vi "calc power.vi"(11 "Array":dbl[][][](array[numeric])) -> (3 "power":dbl)   [LabVIEW 2015]
panel:
  in  "b":dbl=-4445.0 format="%#_13g"
  in  "k":dbl=0.01138 format="%#_13g"
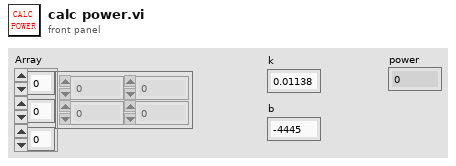
[diagram p1: front panel]
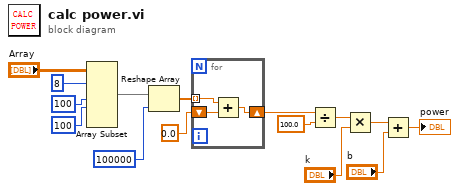
[diagram p0: block diagram]
diagram:
  n1 = Array Subset(array="Array", index (dim 0)=8 ("index"), index (dim 1)=100 ("index"), length (dim 1)=100 ("length")) -> (w1:dbl[][][])  [unwired: 3 in]
  n2 = Reshape Array(w1, 100000 ("dimension size")) -> (w4:dbl[])
  n3 = for {
    tunnel: w4 -> [w18] mode=indexing
    shift-right: [w17] -> w2
    shift-left: 0.0 -> [w16]
    n4 = Add(x=w18, y=w16) -> (x+y=w17:dbl)
  }
  n5 = Divide(x=w2, y=100.0) -> (x/y=w6:dbl)
  n6 = Multiply(x=w6, y="k") -> (x*y=w14:dbl)
  n7 = Add(x=w14, y="b") -> (x+y=→"power":dbl)
